vi "UDP Transfer Group Settings.vi"(8 "error in (no error)":errorcluster, 10 "Transfer Group Configurations":T1[](array[typedef]) {"Transfers"."channels"."dst buffer offset" format="%d bytes"; "Transfers"."channels"."src buffer offset" format="%d bytes"}, 11 "UDP Transceiver in":refnum<class "UDP Transceiver.lvclass">) -> (0 "error out":errorcluster, 3 "UDP Transceiver out":refnum<class "UDP Transceiver.lvclass">)   [LabVIEW 2017, in "UDP.lvlib" / "UDP Transceiver.lvclass"]
uses:
  UDP Transceiver.lvclass
  Builds/Data Sharing Framework/Current/Data Sharing Framework Core/DSF Core.lvlibp/DSF Configuration API/Public/Controls/DSF Engine Transfer Group Configuration.ctl
  Builds/Data Sharing Framework/Current/Data Sharing Framework Core/DSF Core.lvlibp/DSF Configuration API/Public/Controls/DSF Direction.ctl
  Builds/Data Sharing Framework/Current/Data Sharing Framework Core/DSF Core.lvlibp/DSF Configuration API/Public/Controls/DSF Timing Info.ctl
  Builds/Data Sharing Framework/Current/Data Sharing Framework Core/DSF Core.lvlibp/DSF Configuration API/Public/Controls/DSF Engine Transfer Configuration.ctl
  Builds/Data Sharing Framework/Current/Data Sharing Framework Core/DSF Core.lvlibp/DSF Configuration API/Public/Controls/DSF Byte Order.ctl
  Builds/Data Sharing Framework/Current/Data Sharing Framework Core/DSF Core.lvlibp/DSF Configuration API/Public/Controls/DSF Engine Channel Configuration.ctl
  Builds/Data Sharing Framework/Current/Data Sharing Framework Core/DSF Core.lvlibp/DSF Configuration API/Public/Controls/DSF Data Type.ctl
  Builds/Data Sharing Framework/Current/Data Sharing Framework Core/DSF Core.lvlibp/DSF Configuration API/Public/Controls/DSF Settings Info.ctl
  UDP Transceiver.lvclass/UDP Transceiver.ctl
  Transfer Group Parameters.ctl
  Transfer Group Rx Parameters.ctl
  Transfer Rx Parameters.ctl
  Transfer Group Tx Parameters.ctl
  Transfer Tx Parameters.ctl
  Builds/Data Sharing Framework/Current/Data Sharing Framework Core/DSF Core.lvlibp/DSF Configuration API/Public/Required Buffer Size (Transfer).vi
  Builds/Data Sharing Framework/Current/Data Sharing Framework Core/DSF Core.lvlibp
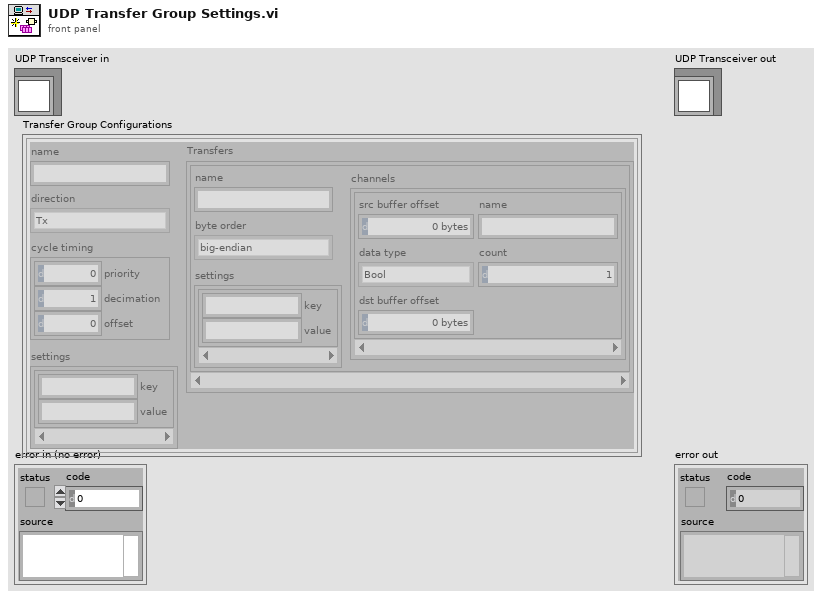
[diagram p1: front panel]
types:
  T1 = typedef "DSF Core.lvlibp/DSF Engine Transfer Group Configuration.ctl" = cluster{"name":string, "direction":T2, "cycle timing":T3, "Transfers":T4[], "settings":T8}
  T2 = typedef "DSF Core.lvlibp/DSF Direction.ctl" = enum8{"Tx", "Rx"}
  T3 = typedef "DSF Core.lvlibp/DSF Timing Info.ctl" = cluster{"priority":u64, "decimation":u64, "offset":u64}
  T4 = typedef "DSF Core.lvlibp/DSF Engine Transfer Configuration.ctl" = cluster{"name":string, "byte order":T5, "channels":T6[], "settings":T8}
  T5 = typedef "DSF Core.lvlibp/DSF Byte Order.ctl" = enum8{"big-endian", "little-endian"}
  T6 = typedef "DSF Core.lvlibp/DSF Engine Channel Configuration.ctl" = cluster{"src buffer offset":u64, "name":string, "data type":T7, "count":u64, "dst buffer offset":u64}
  T7 = typedef "DSF Core.lvlibp/DSF Data Type.ctl" = enum8{"Bool", "SGL", "DBL", "I8", "I16", "I32", "I64", "U8", "U16", "U32", "U64"}
  T8 = typedef "DSF Core.lvlibp/DSF Settings Info.ctl" = cluster{"key":string, "value":string}[]
  T9 = typedef "UDP.lvlib/UDP Transceiver.lvclass/Transfer Group Parameters.ctl" = cluster{"Rx":T10, "Tx":T12}
  T10 = typedef "UDP.lvlib/UDP Transceiver.lvclass/Transfer Group Rx Parameters.ctl" = cluster{"Transfers Rx":T11[], "max size":i32}
  T11 = typedef "UDP.lvlib/UDP Transceiver.lvclass/Transfer Rx Parameters.ctl" = cluster{"timeout":i32, "source address":u32, "source port":u16}
  T12 = typedef "UDP.lvlib/UDP Transceiver.lvclass/Transfer Group Tx Parameters.ctl" = cluster{"Transfers Tx":T13[]}
  T13 = typedef "UDP.lvlib/UDP Transceiver.lvclass/Transfer Tx Parameters.ctl" = cluster{"destination port":u16, "destination address":u32}
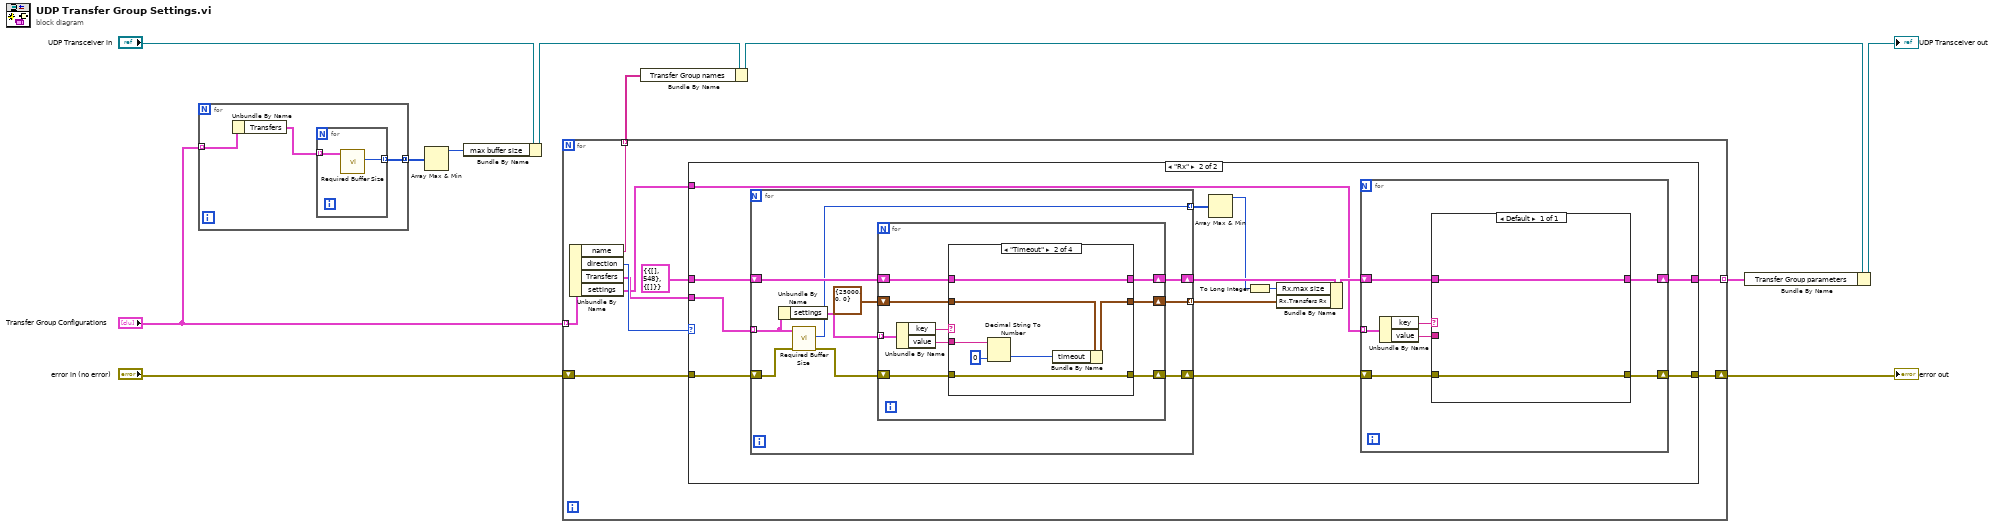
[diagram p0: block diagram]
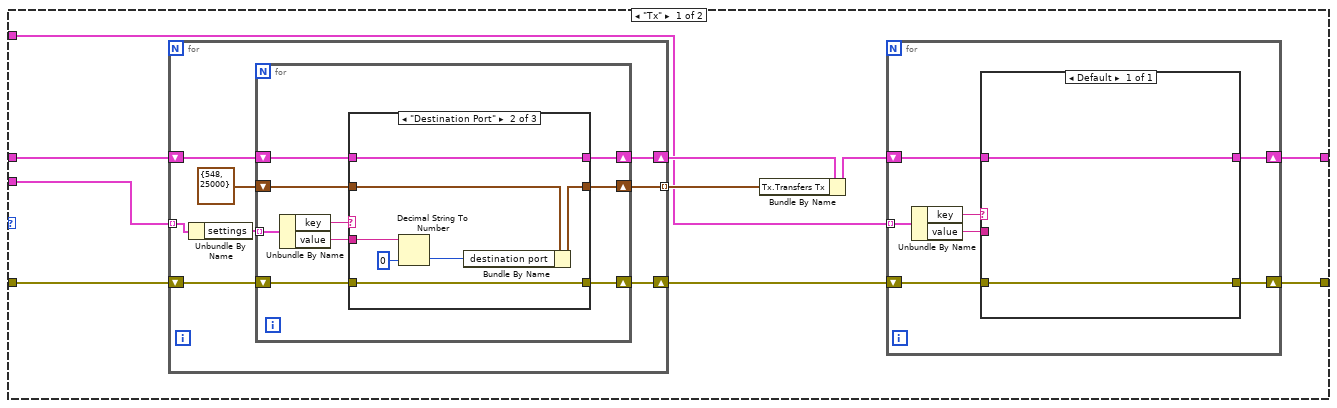
[diagram p2: hidden frame]
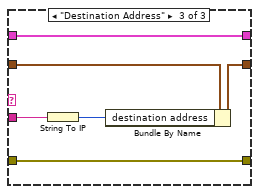
[diagram p4: hidden frame]
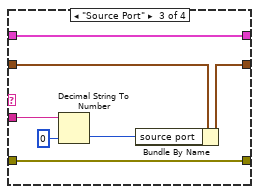
[diagram p6: hidden frame]
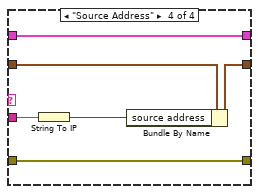
[diagram p7: hidden frame]
diagram:
  n1 = for {
    tunnel: "Transfer Group Configurations" -> [w13] mode=indexing
    tunnel: [w14] -> w11 mode=concatenating
    n2 = Unbundle By Name(w13) -> ("Transfers"=w12:T4[])
    n3 = for {
      tunnel: w12 -> [w16] mode=indexing
      tunnel: [w15] -> w14 mode=indexing
      n4 = call-poly "Required Buffer Size.vi"("Transfer Configuration in"=w16) -> ("required buffer size"=w15:u64)  [unwired: 8 in, 2 out]
    }
  }
  n5 = Array Max & Min(array=w11) -> (max value=w10:u64)  [unwired: 3 out]
  n6 = Bundle By Name(cluster="UDP Transceiver in", "max buffer size"=w10) -> (w9:refnum<class "UDP Transceiver.lvclass">)
  n7 = for {
    tunnel: "Transfer Group Configurations" -> [w21] mode=indexing
    tunnel: [w20] -> w8 mode=indexing
    tunnel: [w25] -> w6 mode=indexing
    shift-right: [w23] -> w1
    shift-left: "error in (no error)" -> [w24]
    n8 = Unbundle By Name(w21) -> ("name"=w20:string, "direction"=w19:T2, "Transfers"=w18:T4[], "settings"=w17:T8)
    n9 = case shown="\"Rx\"" w19 {
      tunnel: T9 {"Rx"={"Transfers Rx"=[], "max size"=548}, "Tx"={"Transfers Tx"=[]}} ("Rx/Tx Parameters") -> [w31 w85]
      tunnel: [w35 w90] -> w25
      tunnel: w24 -> [w33 w86]
      tunnel: [w34 w89] -> w23
      tunnel: w18 -> [w27 w79]
      tunnel: w17 -> [w26 w78]
      frame "Tx" {
        n10 = for {
          shift-right: [w42] -> w30
          shift-left: w31 -> [w43]
          shift-right: [w40] -> w32
          shift-left: w33 -> [w41]
          tunnel: w27 -> [w36] mode=indexing
          tunnel: [w38] -> w29 mode=indexing
          n11 = Unbundle By Name(w36) -> ("settings"=w37:T8)
          n12 = for {
            tunnel: w37 -> [w46] mode=indexing
            shift-right: [w49] -> w42
            shift-left: w43 -> [w50]
            shift-right: [w47] -> w40
            shift-left: w41 -> [w48]
            shift-right: [w45] -> w38
            shift-left: T13 {"destination port"=548, "destination address"=25000} ("Transfer Tx") -> [w44]
            n13 = Unbundle By Name(w46) -> ("key"=w52:string, "value"=w51:string)
            n14 = case shown="\"Destination Port\"" w52 {
              tunnel: w51 -> [_ w62 w67]
              tunnel: w50 -> [w55 w57 w64]
              tunnel: [w55 w57 w64] -> w49
              tunnel: w48 -> [w54 w59 w68]
              tunnel: [w54 w59 w68] -> w47
              tunnel: w44 -> [w53 w58 w65]
              tunnel: [w53 w56 w63] -> w45
              frame Default {
              }
              frame "Destination Port" {
                n15 = Decimal String To Number(string=w62, default (0L)=u16 0 ("default (0 I32)")) -> (number=w60:u16)  [unwired: 1 in, 1 out]
                n16 = Bundle By Name(cluster=w58, "destination port"=w60) -> (w56:T13)
              }
              frame "Destination Address" {
                n17 = String To IP(1:w67) -> (0:w66:u32)
                n18 = Bundle By Name(cluster=w65, "destination address"=w66) -> (w63:T13)
              }
            }
          }
        }
        n19 = Bundle By Name(cluster=w30, "Tx.Transfers Tx"=w29) -> (w28:T9)
        n20 = for {
          tunnel: w26 -> [w73] mode=indexing
          shift-right: [w71] -> w35
          shift-left: w28 -> [w72]
          shift-right: [w69] -> w34
          shift-left: w32 -> [w70]
          n21 = Unbundle By Name(w73) -> ("key"=w75:string, "value"=w74:string)
          n22 = case shown="Default" w75 {
            tunnel: w74 -> [_]
            tunnel: w72 -> [w77]
            tunnel: [w77] -> w71
            tunnel: w70 -> [w76]
            tunnel: [w76] -> w69
            frame Default {
            }
          }
        }
      }
      frame "Rx" {
        n23 = for {
          shift-right: [w99] -> w88
          shift-left: w85 -> [w100]
          shift-right: [w98] -> w83
          shift-left: w86 -> [w92]
          tunnel: w79 -> [w94] mode=indexing
          tunnel: [w96] -> w87 mode=indexing
          tunnel: [w93] -> w82 mode=indexing
          n24 = Unbundle By Name(w94) -> ("settings"=w95:T8)
          n25 = call-poly "Required Buffer Size.vi"("error in (no error)"=w92, "Transfer Configuration in"=w94) -> ("error out"=w91:errorcluster, "required buffer size"=w93:u64)  [unwired: 7 in, 1 out]
          n26 = for {
            tunnel: w95 -> [w103] mode=indexing
            shift-right: [w106] -> w99
            shift-left: w100 -> [w107]
            shift-right: [w104] -> w98
            shift-left: w91 -> [w105]
            shift-right: [w102] -> w96
            shift-left: T11 {"timeout"=25000, "source address"=0, "source port"=0} ("Transfer Rx") -> [w101]
            n27 = Unbundle By Name(w103) -> ("key"=w109:string, "value"=w108:string)
            n28 = case shown="\"Timeout\"" w109 {
              tunnel: w108 -> [_ w119 w126 w128]
              tunnel: w107 -> [w112 w114 w121 w130]
              tunnel: [w112 w114 w121 w130] -> w106
              tunnel: w105 -> [w111 w116 w123 w132]
              tunnel: [w111 w116 w123 w132] -> w104
              tunnel: w101 -> [w110 w115 w122 w131]
              tunnel: [w110 w113 w120 w129] -> w102
              frame Default {
              }
              frame "Timeout" {
                n29 = Decimal String To Number(string=w119, default (0L)=0 ("default (0 I32)")) -> (number=w117:i32)  [unwired: 1 in, 1 out]
                n30 = Bundle By Name(cluster=w115, "timeout"=w117) -> (w113:T11)
              }
              frame "Source Port" {
                n31 = Decimal String To Number(string=w126, default (0L)=u16 0 ("default (0 I32)")) -> (number=w124:u16)  [unwired: 1 in, 1 out]
                n32 = Bundle By Name(cluster=w122, "source port"=w124) -> (w120:T11)
              }
              frame "Source Address" {
                n33 = String To IP(1:w128) -> (0:w127:u32)
                n34 = Bundle By Name(cluster=w131, "source address"=w127) -> (w129:T11)
              }
            }
          }
        }
        n35 = Array Max & Min(array=w82) -> (max value=w81:u64)  [unwired: 3 out]
        n36 = To Long Integer(number=w81) -> (32bit integer=w80:i32)
        n37 = Bundle By Name(cluster=w88, "Rx.max size"=w80, "Rx.Transfers Rx"=w87) -> (w84:T9)
        n38 = for {
          tunnel: w78 -> [w137] mode=indexing
          shift-right: [w135] -> w90
          shift-left: w84 -> [w136]
          shift-right: [w133] -> w89
          shift-left: w83 -> [w134]
          n39 = Unbundle By Name(w137) -> ("key"=w139:string, "value"=w138:string)
          n40 = case shown="Default" w139 {
            tunnel: w138 -> [_]
            tunnel: w136 -> [w141]
            tunnel: [w141] -> w135
            tunnel: w134 -> [w140]
            tunnel: [w140] -> w133
            frame Default {
            }
          }
        }
      }
    }
  }
  "error out" <- w1
  n41 = Bundle By Name(cluster=w9, "Transfer Group names"=w8) -> (w7:refnum<class "UDP Transceiver.lvclass">)
  n42 = Bundle By Name(cluster=w7, "Transfer Group parameters"=w6) -> (→"UDP Transceiver out":refnum<class "UDP Transceiver.lvclass">)
